vi "Main_24B.vi"() -> ()   [LabVIEW 2024]
uses:
  Cluster_Function.ctl
  ENUM_Operand.ctl
  <vilib>/Utility/error.llb/Trim Whitespace One-Sided.vi
  Utility/Universal Utility/TypeDefs_Utility/Cluster_Row-Column.ctl
  9e3f57c0-2ef8-4495-8287-c6a42a5fb955.vi
  Utility/Universal Utility/TypeDefs_Utility/ENUM_4 Directions U-D-L-R.ctl
  Utility/Universal Utility/TypeDefs_Utility/ENUM_8 Directions U-D-L-R.ctl
panel:
  out "Array 2":bool[](array[boolean])
  out "Map 2":map{string, bool}(c390)
  out "Wire Count":i32
  out "Array":T1[](array[typedef])
  out "Map":map{string, bool}(c390)
  in  "Select Data":enum32{"Example", "Example 2", "Puzzle"}(tab)
  in  "Example":string="x00: 1\nx01: 1\nx02: 1\ny00: 0\ny01: 1\ny02: 0\n\nx00 AND y00 -> z00\nx01 XOR y01 -> z01\nx02 OR y02 -> z02"
  in  "Example 2":string="x00: 1\nx01: 0\nx02: 1\nx03: 1\nx04: 0\ny00: 1\ny01: 1\ny02: 1\ny03: 1\ny04: 1\n\nntg XOR fgs -> mjb\ny02 OR x01 -> tnw\nkwq OR kpj -> z05\nx00 OR x03 -> fst\ntgd XOR rvg -> z01\nvdt OR tnw -> bfw\nbfw AND frj -> z10\nffh OR nrd -> bqk\ny00 AND y03 -> djm\ny03 OR y00 -> psh\nbqk OR frj -> z08\ntnw OR fst -> frj\ngnj AND tgd -> z11\nbfw XOR mjb -> z00\nx03 OR x00 -> vdt\ngnj AND wpb -> z02\nx04 AND y00 -> kjc\ndjm OR pbm -> qhw\nnrd AND vdt -> hwm\nkjc AND fst -> rvg\ny04 OR y02 -> fgs\ny01 AND x02 -> pbm\nntg OR kjc -> kwq\npsh XOR fgs -> tgd\nqhw XOR tgd -> z09\npbm OR djm -> kpj\nx03 XOR y03 -> ffh\nx00 XOR y04 -> ntg\nbfw OR bqk -> z06\nnrd XOR fgs -> wpb\nfrj XOR qhw -> z04\nbqk OR frj -> z07\ny03 OR x01 -> nrd\nhwm AND bqk -> z03\ntgd XOR rvg -> z12\ntnw OR pbm -> gnj"
  in  "Puzzle":string="x00: 1\nx01: 0\nx02: 1\nx03: 1\nx04: 0\nx05: 0\nx06: 1\nx07: 1\nx08: 0\nx09: 1\nx10: 1\nx11: 1\nx12: 1\nx13: 1\nx14: 1\nx15: 0\nx16: 1\nx17: 0\nx18: 1\nx19: 1\nx20: 0\nx21: 0\nx22: 1\nx23: 0\nx24: 1\nx25: 0\nx26: 1\nx27: 0\nx28: 1\nx29: 1\nx30: 0\nx31: 0\nx32: 1\nx33: 1\nx34: 1\nx35: 0\nx36: 1\nx37: 1\nx38: 0\nx39: 0\nx40: 1\nx41: 1\nx42: 0\nx43: 0\nx44: 1\ny00: 1\ny01: 0\ny02: 0\ny03: 1\ny04: 1\ny05: 0\ny06: 0\ny07: 0\ny08: 0\ny09: 0\ny10: 0\ny11: 1\ny12: 0\ny13: 0\ny14: 1\ny15: 1\ny16: 0\ny17: 0\ny18: 1\ny19: 0\ny20: 0\ny21: 0\ny22: 1\ny23: 1\ny24: 0\ny25: 0\ny26: 0\ny27: 1\ny28: 1\ny29: 1\ny30: 0\ny31: 1\ny32: 1\ny33: 0\ny34: 1\ny35: 1\ny36: 0\ny37: 0\ny38: 1\ny39: 1\ny40: 1\ny41: 0\ny42: 0\ny43: 1\ny44: 1\n\nnjs AND pvb -> fjh\ny12 AND x12 -> dcm\nsrv XOR dfc -> z22\nqwb XOR vmp -> z14\nnjs XOR pvb -> z10\ncjn OR dfj -> fgc\nkpp XOR tvh -> z34\ntbq OR rdf -> frv\ny40 AND x40 -> drs\npqh XOR mmh -> z05\nx26 XOR y26 -> jkt\nqqp AND dmw -> kqp\nqsh OR wfw -> qcr\nhvw AND qnn -> vgk\nbkc OR wsq -> ckv\nckv XOR bbh -> z03\nfrj XOR hqq -> z02\nqff OR stw -> wsv\nqpq XOR vnr -> z30\npbk XOR kqc -> z15\nmvp OR pbv -> dbj\nx15 AND y15 -> qsh\nwcs OR cqk -> kpp\nbmr XOR fgc -> z32\ny42 XOR x42 -> qjf\nsrv AND dfc -> rng\nrsq AND nts -> brq\nfhv AND hjw -> wwg\nx06 AND y06 -> phw\nvtf AND gdw -> kpc\nwvv AND wbf -> qdh\ny28 AND x28 -> nhs\ny04 AND x04 -> ttv\ncts XOR bcd -> qqp\nmmh AND pqh -> rkt\nhjw XOR fhv -> z37\njdd AND rbm -> z36\ndrt XOR tpt -> z31\ny20 XOR x20 -> gcf\nx27 AND y27 -> ptf\nqnn XOR hvw -> z41\nx13 AND y13 -> msq\ncbr XOR hjd -> z07\nmkv OR hgp -> z45\ny35 XOR x35 -> spp\nx08 XOR y08 -> nrk\ny03 XOR x03 -> bbh\nfhc OR ggh -> fwt\nwhj AND vrh -> qpj\nx34 XOR y34 -> tvh\ny43 AND x43 -> mpm\ny15 XOR x15 -> pbk\nx23 XOR y23 -> bcd\nbwv AND tcd -> sgv\nbcd AND cts -> jcd\nggs OR qmw -> tpt\ngdm XOR jkm -> z09\ny38 XOR x38 -> pgm\nx19 AND y19 -> vmc\ndtc OR ggg -> kqc\nhqq AND frj -> bkc\nsmv OR wwg -> bhh\ny17 AND x17 -> tfq\nx14 AND y14 -> dtc\ny39 AND x39 -> ggh\njmh AND cjc -> gfp\nmgj XOR wsv -> z12\nftd AND wcw -> hjm\ny19 XOR x19 -> whj\nnrk AND ksd -> vwf\nfgq AND spp -> drp\nrsq XOR nts -> z18\ny10 XOR x10 -> njs\nfrv XOR qdb -> z04\nwbk OR fcv -> fgq\nwhj XOR vrh -> z19\ntvh AND kpp -> wbk\ny39 XOR x39 -> pwt\nscg OR gkj -> grv\ndfn XOR qcr -> pbv\nx27 XOR y27 -> ftd\nsvg OR tfq -> rsq\nfkd XOR fwt -> z40\nx07 AND y07 -> pdq\ny13 XOR x13 -> hnt\ngrv XOR vpm -> z21\ny02 XOR x02 -> frj\njkt XOR dbp -> z26\nwdr OR jcd -> z23\nx21 AND y21 -> wns\ny08 AND x08 -> btn\nqqp XOR dmw -> z24\nx01 AND y01 -> wqt\nfrw AND hdp -> hgq\nfrk AND wpk -> hgp\nx07 XOR y07 -> cbr\nx29 AND y29 -> jgm\nsgv OR wqt -> hqq\ntpt AND drt -> dfj\nsdn OR rkt -> kqk\nfrv AND qdb -> vjj\nfjh OR thp -> ncw\ny26 AND x26 -> vvr\nx25 AND y25 -> kcs\nftd XOR wcw -> z27\ntcd XOR bwv -> z01\nbrk XOR kqk -> z06\nx10 AND y10 -> thp\nfrw XOR hdp -> z25\npgm AND bhh -> hsh\nx24 XOR y24 -> dmw\nvmc OR qpj -> bkv\nx44 AND y44 -> mkv\nknh OR vgk -> rps\ndfn AND qcr -> mvp\ntqj OR rng -> cts\ntbb OR wns -> srv\nmsq OR pjj -> vmp\ndrs OR ghn -> hvw\nhsh OR rrb -> rms\ndbj XOR bgt -> z17\nmpm OR kpc -> frk\nbgt AND dbj -> svg\nx40 XOR y40 -> fkd\nx16 AND y16 -> z16\ncbr AND hjd -> dvs\nfsb OR drv -> gdw\ncjc XOR jmh -> z29\npdq OR dvs -> ksd\nrpw OR fbq -> fhv\ny05 XOR x05 -> pqh\nx30 AND y30 -> ggs\nbmb OR drp -> jdd\nhnt XOR fbm -> z13\ny42 AND x42 -> fsb\nqpq AND vnr -> qmw\nx11 XOR y11 -> qff\ngcf AND bkv -> gkj\nwvv XOR wbf -> z28\nx05 AND y05 -> sdn\npqp OR phw -> hjd\njdd XOR rbm -> fbq\nnjt OR kqp -> frw\ny00 XOR x00 -> z00\ny31 AND x31 -> cjn\nx32 XOR y32 -> bmr\nx34 AND y34 -> fcv\ny24 AND x24 -> njt\ny06 XOR x06 -> brk\nx12 XOR y12 -> mgj\nckv AND bbh -> tbq\nrps XOR qjf -> z42\nx33 AND y33 -> cqk\ny09 AND x09 -> nhk\ny33 XOR x33 -> mbp\nx04 XOR y04 -> qdb\nx22 AND y22 -> tqj\ny20 AND x20 -> scg\ny01 XOR x01 -> tcd\nfgc AND bmr -> shp\nmbp XOR pnw -> z33\nfrk XOR wpk -> z44\ny43 XOR x43 -> vtf\nx37 XOR y37 -> hjw\ny03 AND x03 -> rdf\nrms XOR pwt -> z39\nbhh XOR pgm -> z38\nspp XOR fgq -> z35\ny22 XOR x22 -> dfc\nqjf AND rps -> drv\nkcs OR hgq -> dbp\ny29 XOR x29 -> cjc\nx25 XOR y25 -> hdp\nhbq OR dcm -> fbm\nbrk AND kqk -> pqp\nqwb AND vmp -> ggg\ngpb OR shp -> pnw\ny02 AND x02 -> wsq\nptf OR hjm -> wvv\nx18 XOR y18 -> nts\nx23 AND y23 -> wdr\nx09 XOR y09 -> jkm\nx36 AND y36 -> rpw\nx32 AND y32 -> gpb\nmbp AND pnw -> wcs\njgm OR gfp -> qpq\nx11 AND y11 -> qnw\nbkv XOR gcf -> z20\nnhk OR ftf -> pvb\ngdw XOR vtf -> z43\nvjj OR ttv -> mmh\nx41 AND y41 -> knh\nncw XOR qnw -> z11\ny28 XOR x28 -> wbf\ny36 XOR x36 -> rbm\nmgj AND wsv -> hbq\nhnt AND fbm -> pjj\nbrq OR bfd -> vrh\nx17 XOR y17 -> bgt\nksd XOR nrk -> z08\nx38 AND y38 -> rrb\nfwt AND fkd -> ghn\nncw AND qnw -> stw\nx18 AND y18 -> bfd\ny00 AND x00 -> bwv\ngdm AND jkm -> ftf\nrms AND pwt -> fhc\nx16 XOR y16 -> dfn\ny37 AND x37 -> smv\nx35 AND y35 -> bmb\ny30 XOR x30 -> vnr\njkt AND dbp -> dbt\ny41 XOR x41 -> qnn\nx31 XOR y31 -> drt\nqdh OR nhs -> jmh\nvwf OR btn -> gdm\ny44 XOR x44 -> wpk\nx14 XOR y14 -> qwb\nx21 XOR y21 -> vpm\npbk AND kqc -> wfw\nvvr OR dbt -> wcw\ngrv AND vpm -> tbb"
  out "Answer":u64
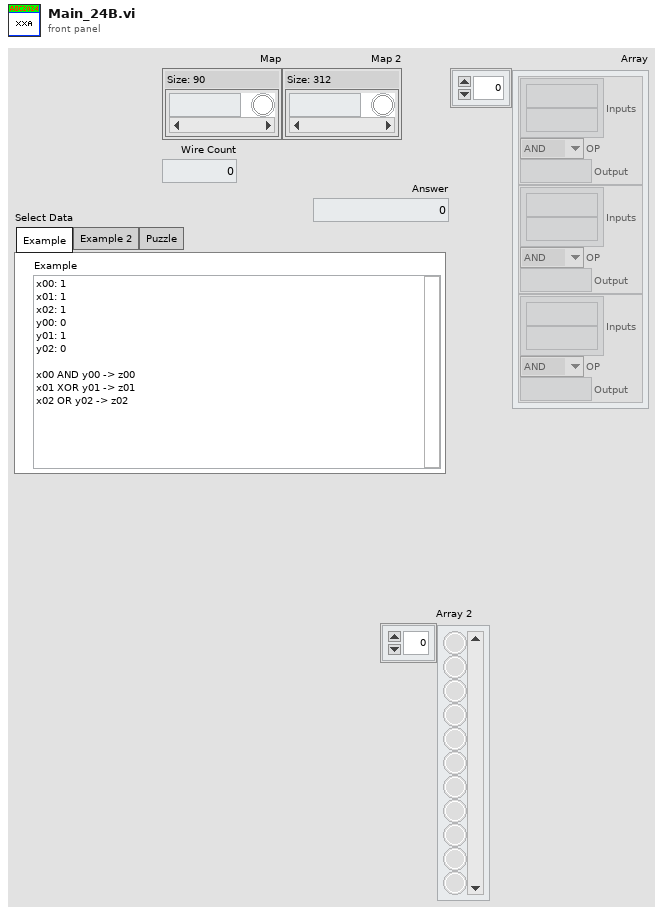
[diagram p1: front panel]
types:
  T1 = typedef "Cluster_Function.ctl" = cluster{"Inputs":string[], "OP":T2, "Output":string}
  T2 = typedef "ENUM_Operand.ctl" = enum16{"AND", "OR", "XOR"}
  T3 = typedef "ENUM_8 Directions U-D-L-R.ctl" = enum16{"Up;-1,0", "Up-Right;-1,1", "Right;0,1", "Down-Right;1,1", "Down;1,0", "Down-Left;1,-1", "Left;0,-1", "Up-Left;-1,-1"}
  T4 = typedef "ENUM_4 Directions U-D-L-R.ctl" = enum16{"Up;-1,0", "Right;0,1", "Down;1,0", "Left;0,-1"}
  T5 = typedef "Cluster_Row-Column.ctl" = cluster{"R":i32, "C":i32}
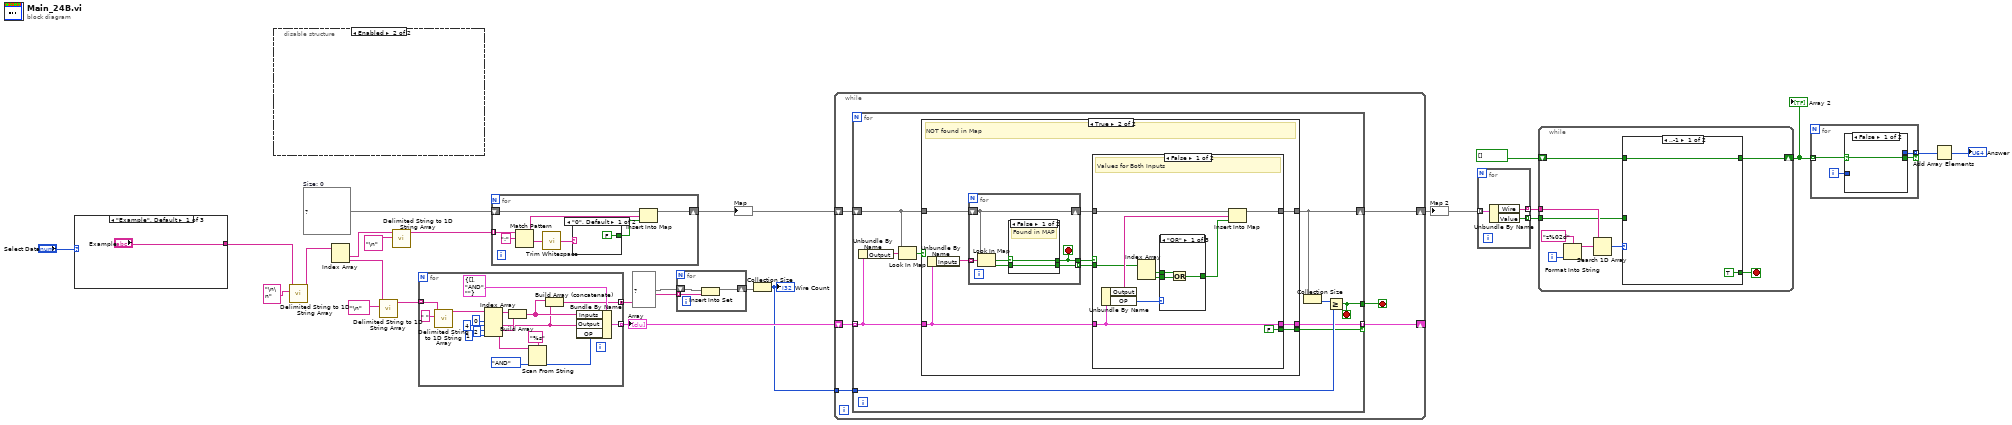
[diagram p0: block diagram]
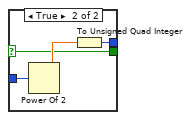
[diagram p2: hidden frame]
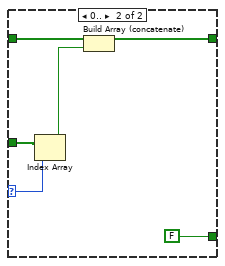
[diagram p3: hidden frame]
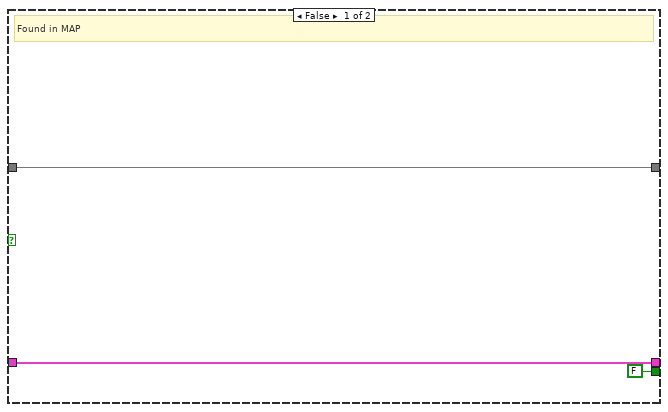
[diagram p4: hidden frame]
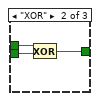
[diagram p5: hidden frame]
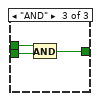
[diagram p6: hidden frame]
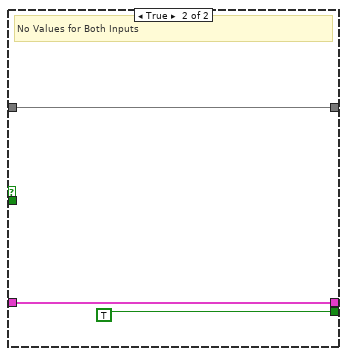
[diagram p7: hidden frame]
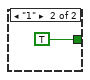
[diagram p9: hidden frame]
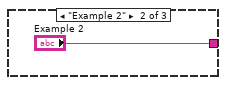
[diagram p10: hidden frame]
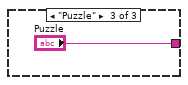
[diagram p11: hidden frame]
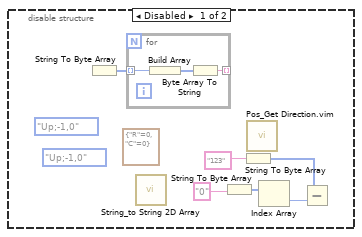
[diagram p12: hidden frame]
diagram:
  w17 = map{string, bool} {}  # Size: 0
  n1 = case shown="\"Example\", Default" "Select Data" {
    tunnel: ["Example" "Example 2" "Puzzle"] -> w22
    frame "Example", Default {
    }
    frame "Example 2" {
    }
    frame "Puzzle" {
    }
  }
  n2 = disable-structure shown="Enabled" {
    frame Disabled {
      (unwired) ENUM_8_Directions_U-D-L-R."Up;-1,0" ("Direction 8")
      (unwired) ENUM_4_Directions_U-D-L-R."Up;-1,0" ("Direction")
      (unwired) T5 {"R"=0, "C"=0} ("Position")
      n3 = String To Byte Array() -> (unsigned byte array=w28:u8[])  [unwired: 1 in]
      n4 = for {
        tunnel: w28 -> [w36] mode=indexing
        tunnel: [w34] -> _ mode=indexing
        n5 = Build Array(w36) -> (w35:u8[])
        n6 = Byte Array To String(unsigned byte array=w35) -> (string=w34:string)
      }
      n7 = call "String_to String 2D Array.vi"() -> ()  [unwired: 11 in, 1 out]
      n8 = String To Byte Array(string="0") -> (unsigned byte array=w31:u8[])
      n9 = String To Byte Array(string="123") -> (unsigned byte array=w29:u8[])
      n10 = call "Pos_Get Direction.vim"() -> ()  [unwired: 11 in, 1 out]
      n11 = Index Array(array=w31) -> (element=w30:u8)  [unwired: 1 in]
      n12 = Subtract(x=w29, y=w30) -> ()  [unwired: 1 out]
    }
    frame Enabled {
    }
  }
  n13 = call <vilib>:"Delimited String to 1D String Array.vi"("delimiter"="\n\n" ("delimiter (Tab)"), "delimited string"=w22) -> ("string array"=w21:string[])  [unwired: 9 in]
  n14 = Index Array(array=w21) -> (element #1=w20:string, element #2=w16:string)  [unwired: 2 in]
  n15 = call <vilib>:"Delimited String to 1D String Array.vi"("delimiter"="\n" ("delimiter (Tab)"), "delimited string"=w16) -> ("string array"=w14:string[])  [unwired: 9 in]
  n16 = call <vilib>:"Delimited String to 1D String Array.vi"("delimiter"="\n" ("delimiter (Tab)"), "delimited string"=w20) -> ("string array"=w18:string[])  [unwired: 9 in]
  n17 = for {
    tunnel: w14 -> [w54] mode=indexing
    tunnel: [w40] -> w10 mode=indexing
    tunnel: [w37] -> w13 mode=concatenating
    n18 = call <vilib>:"Delimited String to 1D String Array.vi"("delimiter"=" ", "delimited string"=w54) -> ("string array"=w52:string[])  [unwired: 9 in]
    n19 = Index Array(array=w52, index #1=0 ("index"), index #2=4 ("index"), index #3=2 ("index"), index #4=1 ("index")) -> (element #1=w47:string, element #2=w38:string, element #3=w46:string, element #4=w44:string)
    n20 = Build Array(w47, w46) -> (w39:string[])
    n21 = Scan From String(format string="%s", input string=w44, default 1=ENUM_Operand."AND" ("OP")) -> (output 1=w41:T2)  [unwired: 2 in, 3 out]
    n22 = Build Array (concatenate)(w39, w38) -> (w37:string[])
    n23 = Bundle By Name(cluster=T1 {"Inputs"=[], "OP"=enum."AND", "Output"=""} ("Function"), "Inputs"=w39, "Output"=w38, "OP"=w41) -> (w40:T1)
  }
  "Array" <- w10
  n24 = for {
    tunnel: w18 -> [w62] mode=indexing
    shift-right: [w59] -> w9
    shift-left: w17 -> [w60]
    n25 = Match Pattern(string=w62, regular expression=":") -> (before substring=w58:string, after substring=w57:string)  [unwired: 1 in, 2 out]
    n26 = call <vilib>:"Trim Whitespace.vi"("string"=w57) -> ("trimmed string"=w56:string)  [unwired: 1 in]
    n27 = case shown="\"0\", Default" w56 {
      tunnel: [FALSE TRUE] -> w55
      frame "0", Default {
      }
      frame "1" {
      }
    }
    n28 = Insert Into Map(map in=w60, key=w58, value=w55) -> (map out=w59:map{string, bool})  [unwired: 2 out]
  }
  "Map" <- w9
  n29 = for {
    tunnel: w13 -> [w67] mode=indexing
    shift-right: [w65] -> w11
    shift-left: set{string} {} ("set in") -> [w66]
    n30 = Insert Into Set(10:w67, 11:w66) -> (3:w65:set{string})  [unwired: 1 out]
  }
  n31 = Collection Size(1:w11) -> (0:w8:i32)
  "Wire Count" <- w8
  n32 = while {
    shift-right: [w71] -> w7
    shift-left: w9 -> [w72]
    tunnel: w8 -> [w70]
    shift-right: [w68] -> _
    shift-left: w10 -> [w73]
    stop <- w69 stop-if-true
    n33 = for {
      tunnel: w73 -> [w76] mode=indexing
      shift-right: [w80] -> w71
      shift-left: w72 -> [w81]
      tunnel: w70 -> [w78]
      tunnel: [w77] -> w69
      tunnel: [w75] -> w68 mode=indexing if=w74
      stop <- w77 stop-if-true
      n34 = Unbundle By Name(w76) -> ("Output"=w83:string)
      n35 = Look In Map(map=w81, key=w83) -> (key not found?=w82:bool)  [unwired: 1 in, 1 out]
      n36 = case shown="True" w82 {
        tunnel: w81 -> [w86 w95]
        tunnel: [w86 w91] -> w80
        tunnel: w76 -> [w85 w90]
        tunnel: [w85 w89] -> w75
        tunnel: [FALSE w88] -> w74
        frame False {
          # "Found in MAP"
        }
        frame True {
          # "NOT found in Map"
          n37 = Unbundle By Name(w90) -> ("Inputs"=w94:string[])
          n38 = for {
            shift-right: [w122] -> w93
            shift-left: w95 -> [w122]
            tunnel: w94 -> [w123] mode=indexing
            tunnel: [w120] -> w87 mode=indexing
            tunnel: [w118] -> w92
            stop <- w118 stop-if-true
            n39 = Look In Map(map=w122, key=w123) -> (key not found?=w121:bool, value=w119:bool)  [unwired: 1 in]
            n40 = case shown="False" w121 {
              selector: w121 -> [w125 w126]
              tunnel: [w125 w126] -> w118
              tunnel: [w124 _] -> w120
              tunnel: w119 -> [w124 _]
              frame False {
                # "Found in MAP"
              }
              frame True {
                # "NOT Found in Map"
              }
            }
          }
          n41 = case shown="False" w92 {
            tunnel: w93 -> [w103 w117]
            tunnel: [w102 w117] -> w91
            tunnel: w90 -> [w104 w116]
            tunnel: [w104 w116] -> w89
            tunnel: [FALSE TRUE] -> w88
            tunnel: w87 -> [w99 _]
            frame False {
              # "Values for Both Inputs"
              n42 = Unbundle By Name(w104) -> ("Output"=w101:string, "OP"=w100:T2)
              n43 = Index Array(array=w99) -> (element #1=w98:bool, element #2=w97:bool)  [unwired: 2 in]
              n44 = case shown="\"OR\"" w100 {
                tunnel: w98 -> [w108 w111 w114]
                tunnel: w97 -> [w107 w110 w113]
                tunnel: [w106 w109 w112] -> w96
                frame "OR" {
                  n45 = Or(x=w108, y=w107) -> (x .or. y?=w106:bool)
                }
                frame "XOR" {
                  n46 = Exclusive Or(1:w110, 2:w111) -> (0:w109:bool)
                }
                frame "AND" {
                  n47 = And(x=w114, y=w113) -> (x .and. y?=w112:bool)
                }
              }
              n48 = Insert Into Map(map in=w103, key=w101, value=w96) -> (map out=w102:map{string, bool})  [unwired: 2 out]
            }
            frame True {
              # "No Values for Both Inputs"
            }
          }
        }
      }
      n49 = Collection Size(1:w80) -> (0:w79:i32)
      n50 = Greater Or Equal?(x=w79, y=w78) -> (x >= y?=w77:bool)
    }
  }
  "Map 2" <- w7
  n51 = for {
    tunnel: w7 -> [w129] mode=indexing
    tunnel: [w128] -> w6 mode=indexing
    tunnel: [w127] -> w5 mode=indexing
    n52 = Unbundle By Name(w129) -> ("Wire"=w128:string, "Value"=w127:bool)
  }
  n53 = while {
    tunnel: w6 -> [w136]
    tunnel: w5 -> [w130]
    shift-right: [w131] -> w3
    shift-left: bool[] [] -> [w133]
    i -> [w138]
    stop <- w132 stop-if-true
    n54 = Format Into String(format string="z%02d", w138) -> (resulting string=w135:string)  [unwired: 2 in, 1 out]
    n55 = Search 1D Array(1D array=w136, element=w135) -> (index of element=w134:i32)  [unwired: 1 in]
    n56 = case shown="..-1" w134 {
      selector: w134 -> [_ w142]
      tunnel: w133 -> [w140 w145]
      tunnel: [TRUE FALSE] -> w132
      tunnel: [w140 w144] -> w131
      tunnel: w130 -> [_ w143]
      frame ..-1 {
      }
      frame 0.. {
        n57 = Index Array(array=w143, index=w142) -> (element=w141:bool)
        n58 = Build Array (concatenate)(w145, w141) -> (w144:bool[])
      }
    }
  }
  "Array 2" <- w3
  n59 = for {
    tunnel: w3 -> [w149] mode=indexing
    tunnel: [w148] -> w2 mode=indexing if=w147
    i -> [w150]
    n60 = case shown="False" w149 {
      selector: w149 -> [w151 w153]
      tunnel: w150 -> [_ w155]
      tunnel: [w151 w153] -> w147
      tunnel: [_ w152] -> w148
      frame False {
      }
      frame True {
        n61 = Power Of 2(x=w155) -> (2^x=w154:dbl)
        n62 = To Unsigned Quad Integer(1:w154) -> (0:w152:u64)
      }
    }
  }
  n63 = Add Array Elements(numeric array=w2) -> (sum=→"Answer":u64)
